vi "Write Data.vi"(0 "comm interface in":refnum<class "RoboRIO UART.lvclass">, 5 "data":u8[](array[numeric]), 11 "error in":errorcluster) -> (4 "comm interface out":refnum<class "RoboRIO UART.lvclass">, 15 "error out":errorcluster)   [LabVIEW 2018, in "RoboRIO UART.lvclass"]
uses:
  RoboRIO UART.lvclass
  RoboRIO UART.lvclass/RoboRIO UART.ctl
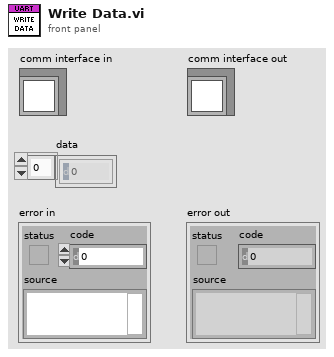
[diagram p1: front panel]
types:
  T1 = typedef "WPI_SerialPortRef.ctl" = cluster{"DevStatus":errorcluster, "Serial Port Name":refnum<visa-resource-name>}
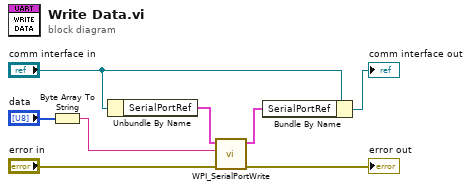
[diagram p0: block diagram]
diagram:
  n1 = Byte Array To String(unsigned byte array="data") -> (string=w1:string)
  n2 = Unbundle By Name("comm interface in") -> ("SerialPortRef"=w5:T1)
  n3 = call <vilib>:"WPI_SerialPortWrite.vi"("error in (no error)"="error in", "Buffer"=w1, "SerialPortRef"=w5) -> ("error out"=→"error out":errorcluster, "SerialPortRef"=w6:T1)  [unwired: 6 in, 1 out]
  n4 = Bundle By Name(cluster="comm interface in", "SerialPortRef"=w6) -> (→"comm interface out":refnum<class "RoboRIO UART.lvclass">)
